vi "Ctor.vi"(8 "error in (no error)":errorcluster, 11 "Tester in":refnum<class "Tester.lvclass">) -> (0 "error out":errorcluster, 3 "Tester out":refnum<class "Tester.lvclass">)   [LabVIEW 2020, in "Tester.lvlib" / "Tester.lvclass"]
uses:
  Tester.lvclass
  Config Ref.ctl
  Execution Ref.ctl
  Sequence/Sequence.lvclass
  Results/Results.lvclass
  State.ctl
  Tester.lvclass/Tester.ctl
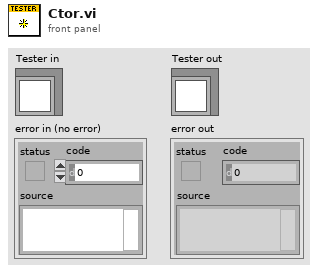
[diagram p1: front panel]
types:
  T1 = typedef "Tester.lvlib/Tester.lvclass/Execution Ref.ctl" = cluster{"Sequence":refnum<class "Sequence.lvclass">, "Step":i32, "Results":refnum<class "Results.lvclass">, "State":T2, "Run Step VI":refnum<vi>, "Abort":bool}
  T2 = typedef "Tester.lvlib/Tester.lvclass/State.ctl" = enum16{"Idle", "In Progress", "Completed"}
  T3 = typedef "Tester.lvlib/Tester.lvclass/Config Ref.ctl" = cluster{"Stop on Fail":bool, "Stop on Error":bool}
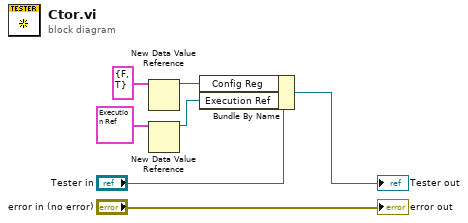
[diagram p0: block diagram]
diagram:
  n1 = New Data Value Reference(data value=T3 {"Stop on Fail"=FALSE, "Stop on Error"=TRUE} ("Config Ref")) -> (data value reference=w2:refnum<data-value>)  [unwired: 1 in, 1 out]
  n2 = New Data Value Reference(data value=T1 {"Sequence"=refnum, "Step"=0, "Results"=refnum, "State"=enum."Idle", "Run Step VI"=refnum, "Abort"=FALSE} ("Execution Ref")) -> (data value reference=w1:refnum<data-value>)  [unwired: 1 in, 1 out]
  n3 = Bundle By Name(cluster="Tester in", "Config Reg"=w2, "Execution Ref"=w1) -> (→"Tester out":refnum<class "Tester.lvclass">)
  "error out" <- "error in (no error)"
